vi "pdw 2 raw PDWs.vi"(8 "error in (no error)":errorcluster, 10 "PDWs":T1[](array[typedef]), 11 "device_type in":refnum<class "device_type.lvclass">) -> (0 "error out":errorcluster, 2 "Array":u64[][](array[numeric]), 3 "device_type out":refnum<class "device_type.lvclass">)   [LabVIEW 2021, in "device_type.lvclass"]
uses:
  device_type.lvclass
  pulse_tx_vis/CTL/PDW_lv2.ctl
  pulse_tx_vis/CTL/mode_type.ctl
  device_type.lvclass/device_type.ctl
  pulse_tx_vis/pdw.ctl
panel:
  out "lfm lost":bool
  out "mod too wide":bool
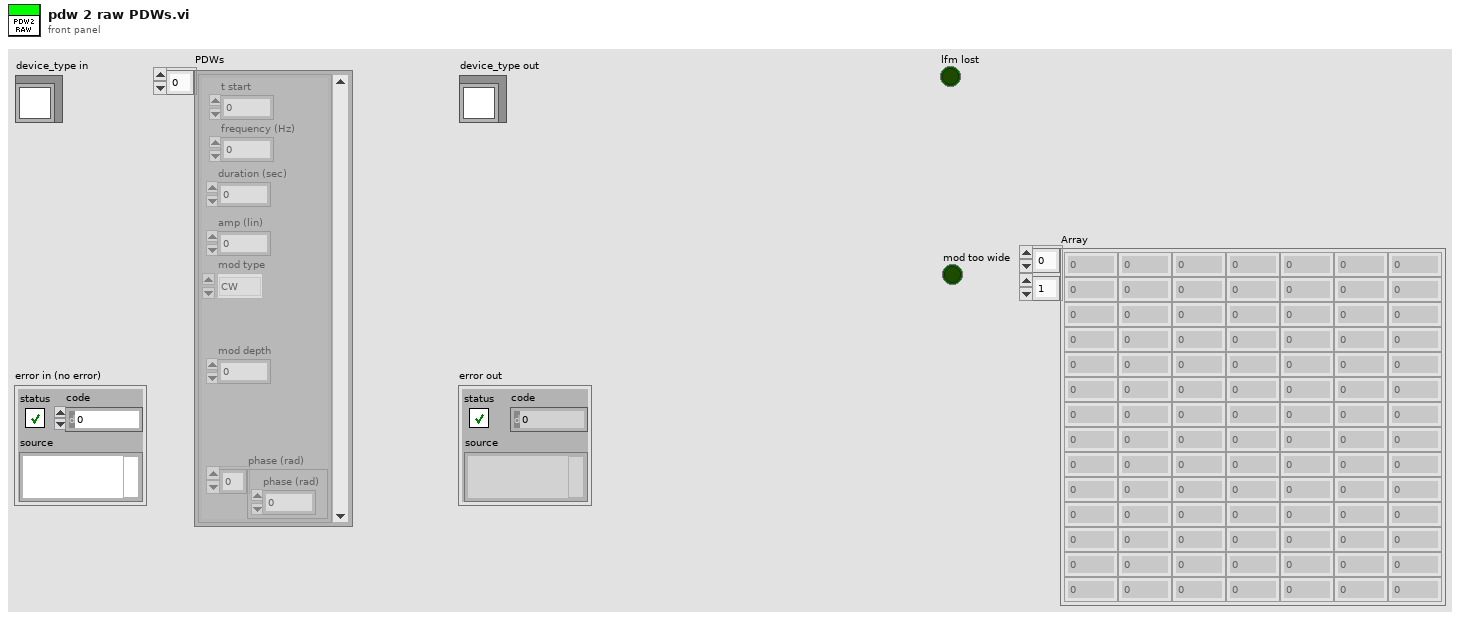
[diagram p1: front panel]
types:
  T1 = typedef "PDW_lv2.ctl" = cluster{"t start":dbl, "frequency (Hz)":dbl, "duration (sec)":dbl, "amp (lin)":dbl, "mod type":T2, "mod depth":dbl, "phase (rad)":dbl[]}
  T2 = typedef "mode_type.ctl" = enum8{"CW", "from memory 1", "NC - cw", "LFM", "BPSK", "QPSK"}
  T3 = typedef "pdw.ctl" = cluster{"PW":u32, "frequency shift":fxp<+/-,48,0>, "amp":fxp<+/-,18,1>, "mode type":T2, "mode depth":u32, "mode filter":u8, "phase shift":fxp<+/-,16,1>, "pulse shape filter":u8}
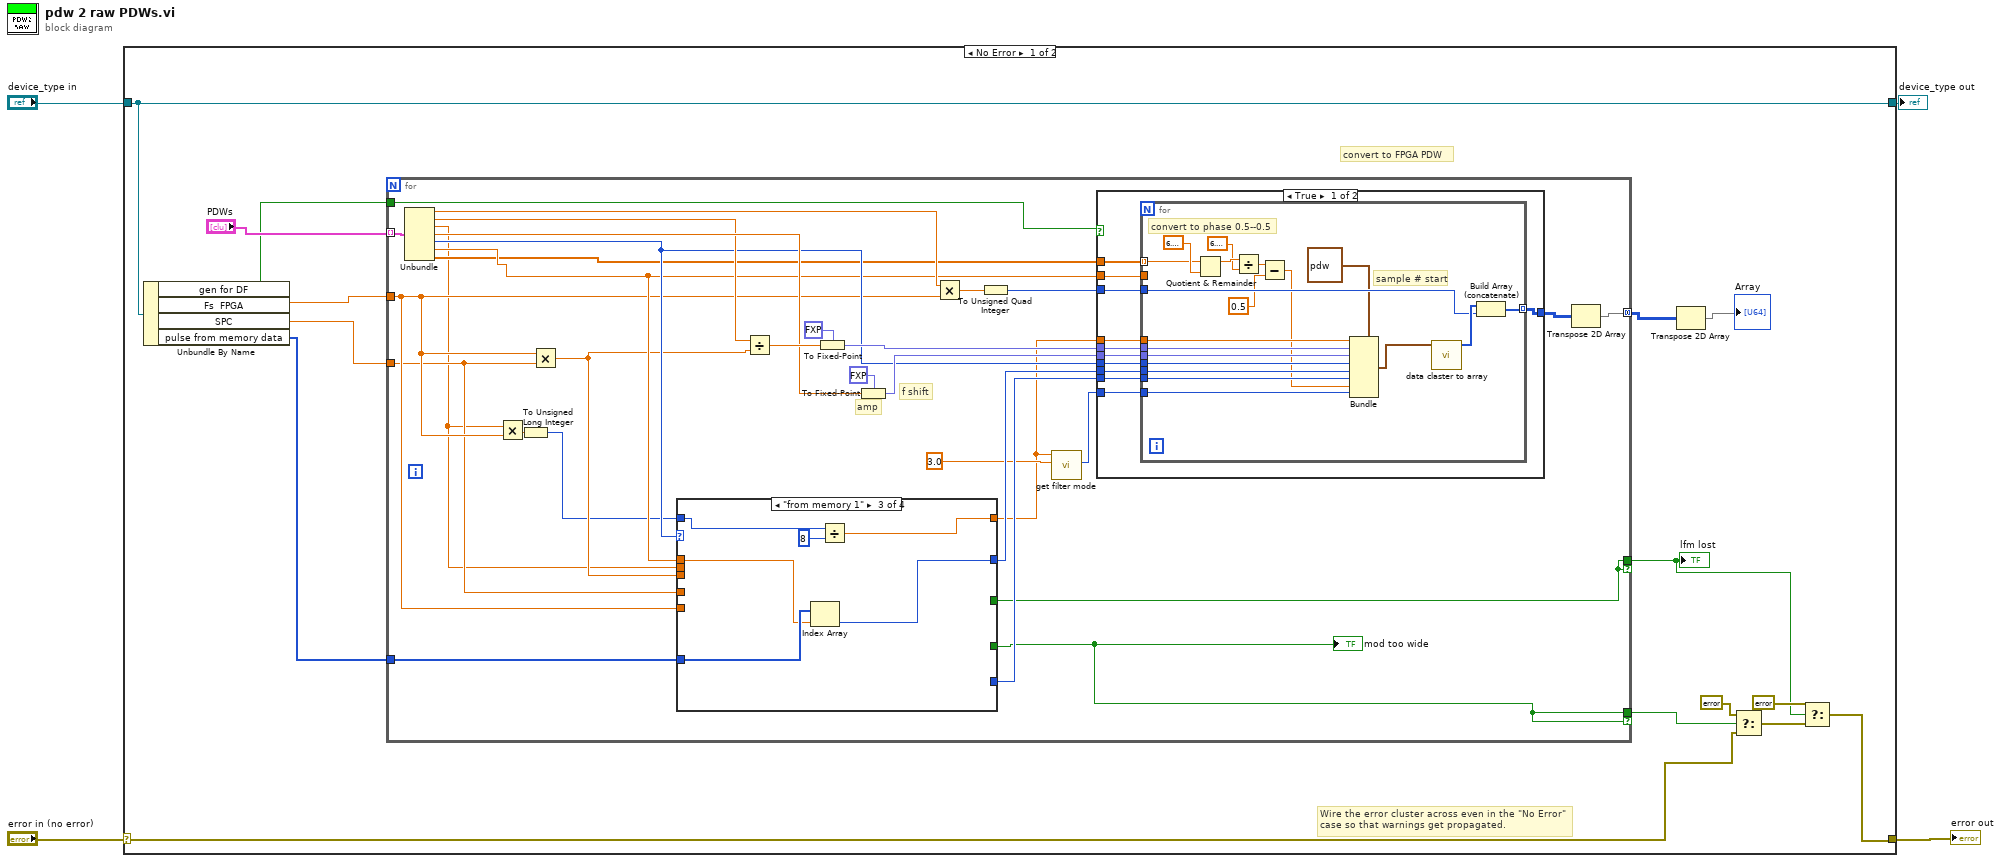
[diagram p0: block diagram]
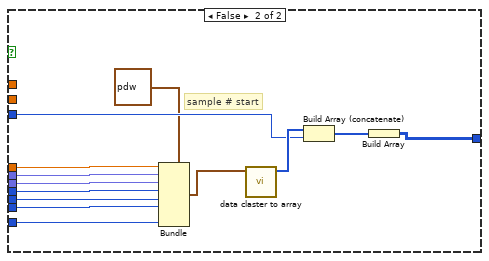
[diagram p2: hidden frame]
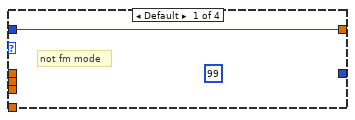
[diagram p3: hidden frame]
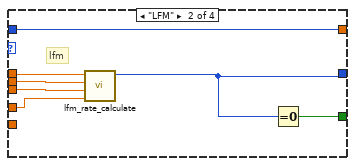
[diagram p4: hidden frame]
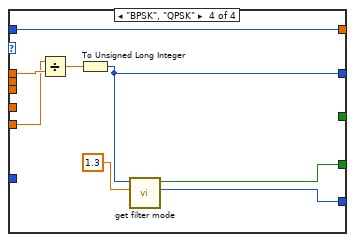
[diagram p5: hidden frame]
diagram:
  n1 = case shown="No Error" "error in (no error)" {
    selector: "error in (no error)" -> [w8 w117]
    tunnel: [w7 w117] -> w3
    tunnel: [w11 w116] -> w1
    tunnel: "device_type in" -> [w11 w116]
    frame No Error {
      # "convert to FPGA PDW"
      # "Wire the error cluster across even in the \"No Error\"\ncase so that warnings get propagated."
      n2 = Unbundle By Name(w11) -> ("gen for DF"=w6:bool, "Fs  FPGA"=w10:dbl, "SPC"=w9:dbl, "pulse from memory data"=w5:u32[])
      n3 = for {
        tunnel: "PDWs" -> [w50] mode=indexing
        tunnel: [w33] -> w14 mode=concatenating
        tunnel: w10 -> [w28]
        tunnel: [w30] -> w12 if=w30
        tunnel: [w35] -> w17 if=w35
        tunnel: w9 -> [w27]
        tunnel: w6 -> [w24]
        tunnel: w5 -> [w20]
        # "amp"
        # "f shift"
        n4 = Unbundle(w50) -> ("t start"=w49:dbl, "frequency (Hz)"=w39:dbl, "duration (sec)"=w22:dbl, "amp (lin)"=w43:dbl, "mod type"=w38:T2, "mod depth"=w32:dbl, "phase (rad)"=w31:dbl[])
        n5 = Multiply(x=w22, y=w28) -> (x*y=w44:dbl)
        n6 = To Unsigned Long Integer(number=w44) -> (unsigned 32bit integer=w23:u32)
        n7 = Multiply(x=w28, y=w27) -> (x*y=w29:dbl)
        n8 = case shown="\"from memory 1\"" w38 {
          tunnel: [_ w98 w102 w112] -> w37
          tunnel: w29 -> [_ w101 _ _]
          tunnel: w32 -> [_ w99 w106 w115]
          tunnel: w22 -> [_ w100 _ _]
          tunnel: [_ _ _ w113] -> w36
          tunnel: [_ _ _ w111] -> w35
          tunnel: [_ w97 _ _] -> w30
          tunnel: w28 -> [_ _ _ w110]
          tunnel: w27 -> [_ w96 _ _]
          tunnel: w23 -> [w94 w95 w105 w108]
          tunnel: [w94 w95 w103 w108] -> w21
          tunnel: w20 -> [_ _ w107 _]
          frame Default {
            (unwired) u32 99 ("integer (fxp cast)")
            # "not fm mode"
          }
          frame "LFM" {
            # "lfm"
            n9 = call "lfm_rate_calculate.vi"("SPC"=w96, "fs"=w101, "pw"=w100, "f span"=w99) -> ("integer (fxp cast)"=w98:u32)  [unwired: 7 in]
            n10 = Equal To 0?(x=w98) -> (x = 0?=w97:bool)
          }
          frame "from memory 1" {
            n11 = Index Array(array=w107, index=w106) -> (element=w102:u32)
            n12 = Divide(x=w105, y=u32 8) -> (x/y=w103:dbl)
          }
          frame "BPSK", "QPSK" {
            n13 = Divide(x=w110, y=w115) -> (x/y=w114:dbl)
            n14 = To Unsigned Long Integer(number=w114) -> (unsigned 32bit integer=w112:u32)
            n15 = call "get filter mode.vi"("filter rate"=1.3 ("y"), "Numeric in"=w112) -> ("filter mode"=w113:i32, "no fit filter"=w111:bool)  [unwired: 8 in]
          }
        }
        "mod too wide" <- w35
        n16 = Divide(x=w39, y=w29) -> (x/y=w47:dbl)
        n17 = To Fixed-Point(fixed-point type=fxp<+/-,48,0> 0.0 ("frequency shift"), number=w47) -> (fixed-point=w45:fxp<+/-,48,0>)
        n18 = To Fixed-Point(fixed-point type=fxp<+/-,18,1> 0.0 ("I"), number=w43) -> (fixed-point=w41:fxp<+/-,18,1>)
        n19 = Multiply(x=w49, y=w28) -> (x*y=w48:dbl)
        n20 = To Unsigned Quad Integer(1:w48) -> (0:w40:u64)
        n21 = call "get filter mode.vi"("filter rate"=3.0, "Numeric in"=w21) -> ("filter mode"=w25:i32)  [unwired: 8 in, 1 out]
        n22 = case shown="True" w24 {
          tunnel: w45 -> [w61 w93]
          tunnel: w41 -> [w60 w92]
          tunnel: w40 -> [w59 w90]
          tunnel: [w58 w83] -> w34
          tunnel: w21 -> [w57 w87]
          tunnel: w38 -> [w56 w86]
          tunnel: w37 -> [w55 w82]
          tunnel: w36 -> [w54 w85]
          tunnel: w32 -> [w53 _]
          tunnel: w31 -> [w52 _]
          tunnel: w25 -> [w51 w81]
          frame True {
            n23 = for {
              tunnel: w61 -> [w80]
              tunnel: w60 -> [w79]
              tunnel: w59 -> [w77]
              tunnel: [w74] -> w58 mode=indexing
              tunnel: w57 -> [w73]
              tunnel: w56 -> [w72]
              tunnel: w55 -> [w71]
              tunnel: w54 -> [w70]
              tunnel: w53 -> [_]
              tunnel: w52 -> [w63] mode=indexing
              tunnel: w51 -> [w62]
              # "convert to phase 0.5--0.5"
              # "sample # start"
              n24 = Quotient & Remainder(x=w63, y=6.283185307179586) -> (x-y*floor(x/y)=w68:dbl)  [unwired: 1 out]
              n25 = Divide(x=w68, y=6.283185307179586) -> (x/y=w66:dbl)
              n26 = Subtract(x=w66, y=0.5) -> (x-y=w64:dbl)
              n27 = Bundle(cluster=T3 {"PW"=0, "frequency shift"=0.0, "amp"=0.0, "mode type"=enum."CW", "mode depth"=0, "mode filter"=0, "phase shift"=0.0, "pulse shape filter"=0} ("Cluster"), "PW"=w73, "frequency shift"=w80, "amp"=w79, "mode type"=w72, "mode depth"=w71, "mode filter"=w70, "phase shift"=w64, "pulse shape filter"=w62) -> (w75:T3)
              n28 = call "data claster to array.vi"("Cluster"=w75) -> ("Array"=w78:u64[])  [unwired: 10 in]
              n29 = Build Array (concatenate)(w78, w77) -> (w74:u64[])
            }
          }
          frame False {
            # "sample # start"
            n30 = Bundle(cluster=T3 {"PW"=0, "frequency shift"=0.0, "amp"=0.0, "mode type"=enum."CW", "mode depth"=0, "mode filter"=0, "phase shift"=0.0, "pulse shape filter"=0} ("Cluster"), "PW"=w87, "frequency shift"=w93, "amp"=w92, "mode type"=w86, "mode depth"=w82, "mode filter"=w85, "pulse shape filter"=w81) -> (w88:T3)  [unwired: 1 in]
            n31 = call "data claster to array.vi"("Cluster"=w88) -> ("Array"=w91:u64[])  [unwired: 10 in]
            n32 = Build Array (concatenate)(w91, w90) -> (w84:u64[])
            n33 = Build Array(w84) -> (w83:u64[][])
          }
        }
        n34 = Transpose 2D Array(2D array=w34) -> (transposed array=w33:u64[][])
      }
      "lfm lost" <- w12
      n35 = Transpose 2D Array(2D array=w14) -> (transposed array=→"Array":u64[][])
      n36 = Select(t=errorcluster {"status"=TRUE, "code"=5432, "source"="PSK mod too wide"} ("error out"), s=w17, f=w8) -> (s? t:f=w16:errorcluster)
      n37 = Select(t=errorcluster {"status"=TRUE, "code"=5432, "source"="The LFM value lost, pls take higher value for it"} ("error out"), s=w12, f=w16) -> (s? t:f=w7:errorcluster)
    }
    frame Error {
    }
  }
  "error out" <- w3
  "device_type out" <- w1
